vi "Build SeqEdit Execution Plan.vi"(8 "error in":errorcluster, 10 "Environment":path, 11 "TSInstall":T2) -> (0 "error out":errorcluster, 3 "Execution Plan":T1={"Exe Path"=path "", "Args"=[], "Timeout"=-1})   [LabVIEW 2025]
doc: "This VI builds an execution plan to launch the TestStand Sequence Editor with optional environment arguments."
uses:
  Type Definitions/TSInstall--cluster.ctl
  Type Definitions/Architecture--enum.ctl
  Type Definitions/Execution Plan--cluster.ctl
  <userlib>/_OpenG.lib/file/file.llb/Strip Path Extension - Path__ogtk.vi
  <userlib>/_OpenG.lib/file/file.llb/File Exists - Scalar__ogtk.vi
  <userlib>/_OpenG.lib/file/file.llb/openg_file.lvlib
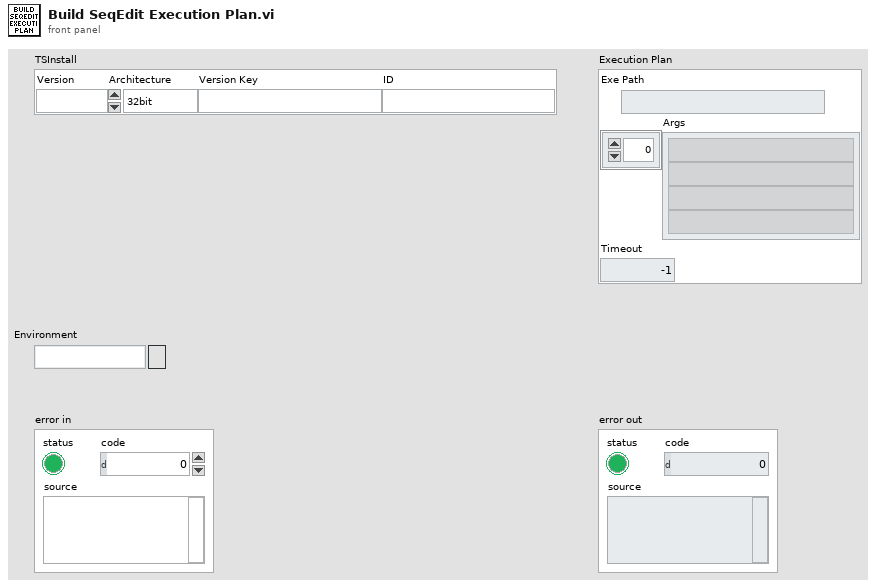
[diagram p1: front panel]
types:
  T1 = typedef "Execution Plan--cluster.ctl" = cluster{"Exe Path":path, "Args":string[], "Timeout":i32}
  T2 = typedef "TSInstall--cluster.ctl" = cluster{"Version":string, "Architecture":T3, "Version Key":string, "ID":string}
  T3 = typedef "Architecture--enum.ctl" = enum16{"32bit", "64bit"}
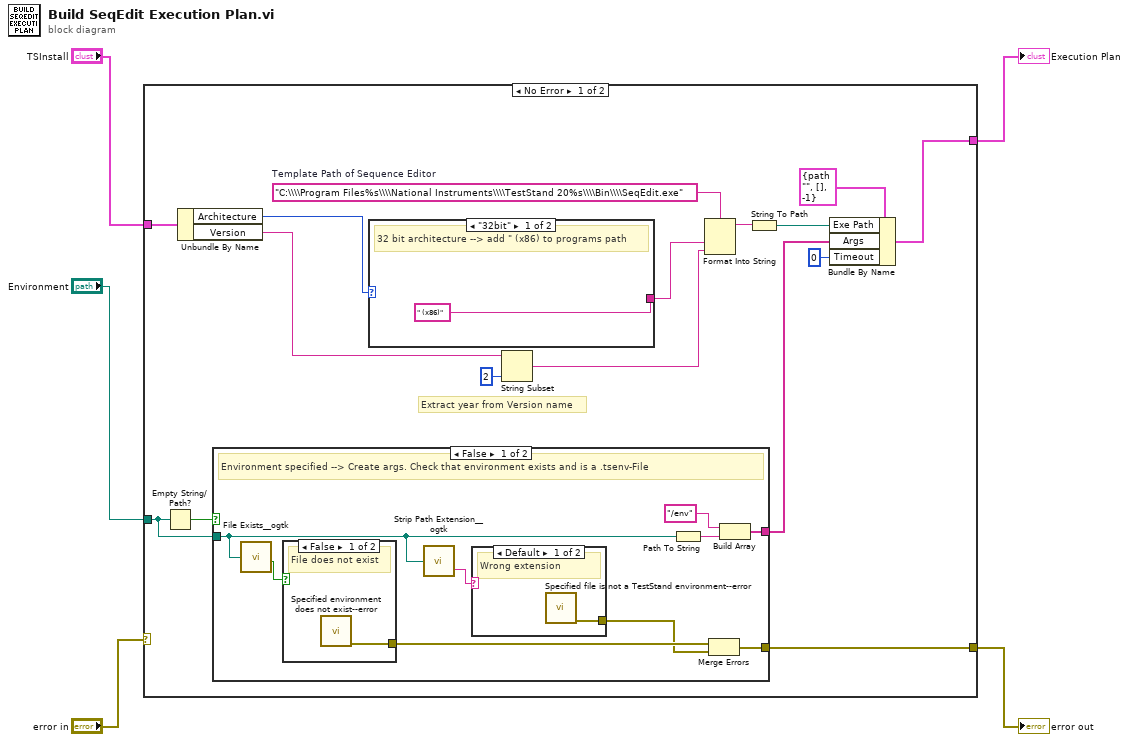
[diagram p0: block diagram]
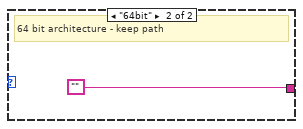
[diagram p5: hidden frame]
diagram:
  n1 = case shown="No Error" "error in" {
    selector: "error in" -> [_ w35]
    tunnel: "TSInstall" -> [w21 _]
    tunnel: [w11 _] -> w4
    tunnel: "Environment" -> [w9 _]
    tunnel: [w6 w35] -> w1
    frame No Error {
      w20 = "C:\\\\Program Files%s\\\\National Instruments\\\\TestStand 20%s\\\\Bin\\\\SeqEdit.exe"  # Template Path of Sequence Editor
      # "Extract year from Version name"
      n2 = Empty String/Path?(string/path=w9) -> (empty?=w10:bool)
      n3 = Unbundle By Name(w21) -> ("Architecture"=w17:T3, "Version"=w18:string)
      n4 = case shown="False" w10 {
        tunnel: w9 -> [w27 _]
        tunnel: [w28 _] -> w8
        tunnel: [w22 _] -> w6
        frame False {
          # "Environment specified --> Create args. Check that environment exists and is a .tsenv-File"
          n5 = call-poly <userlib>:"File Exists__ogtk.vi"("file path"=w27) -> ("exists"=w25:bool)  [unwired: 6 in, 1 out]
          n6 = case shown="False" w25 {
            tunnel: [w31 _] -> w24
            frame False {
              # "File does not exist"
              n7 = call "Specified environment does not exist--error.vi"() -> ("error out"=w31:errorcluster)  [unwired: 11 in]
            }
            frame True {
              # "File exists"
            }
          }
          n8 = call-poly <userlib>:"Strip Path Extension__ogtk.vi"("path"=w27) -> ("extension"=w26:string)  [unwired: 1 out]
          n9 = case shown="Default" w26 {
            tunnel: [w32 _] -> w23
            frame Default {
              # "Wrong extension"
              n10 = call "Specified file is not a TestStand environment--error.vi"() -> ("error out"=w32:errorcluster)  [unwired: 11 in]
            }
            frame "tsenv" {
              # "Right extension"
            }
          }
          n11 = Path To String(path=w27) -> (string=w29:string)
          n12 = Merge Errors(w24, w23) -> (w22:errorcluster)
          n13 = Build Array("/env", w29) -> (w28:string[])
        }
        frame True {
          # "No environment specified"
        }
      }
      n14 = case shown="\"32bit\"" w17 {
        tunnel: [" (x86)" ""] -> w16
        frame "32bit" {
          # "32 bit architecture --> add \" (x86) to programs path"
        }
        frame "64bit" {
          # "64 bit architecture - keep path"
        }
      }
      n15 = String Subset(string=w18, length (rest)=2 ("length (rest)")) -> (substring=w15:string)  [unwired: 1 in]
      n16 = Format Into String(format string=w20, w16, w15) -> (resulting string=w14:string)  [unwired: 2 in, 1 out]
      n17 = String To Path(string=w14) -> (path=w12:path)
      n18 = Bundle By Name(cluster=T1 {"Exe Path"=path "", "Args"=[], "Timeout"=-1} ("Execution Plan"), "Exe Path"=w12, "Args"=w8, "Timeout"=0) -> (w11:T1)
    }
    frame Error {
      # "Pass error without further action"
    }
  }
  "Execution Plan" <- w4
  "error out" <- w1
